vi "Write System.vi"(8 "error in (no error)":errorcluster, 10 "System":refnum<class "Message Enqueuer.lvclass">, 11 "Command in":refnum<class "Command Actor.lvclass">) -> (0 "error out":errorcluster, 3 "Command out":refnum<class "Command Actor.lvclass">)   [LabVIEW 2014, in "Robot Actor Framework.lvlib" / "Command Actor.lvlib" / "Command Actor.lvclass"]
uses:
  Command Actor.lvclass
  <vilib>/ActorFramework/Message Enqueuer/Message Enqueuer.lvclass
  Command Actor.lvclass/Command Actor.ctl
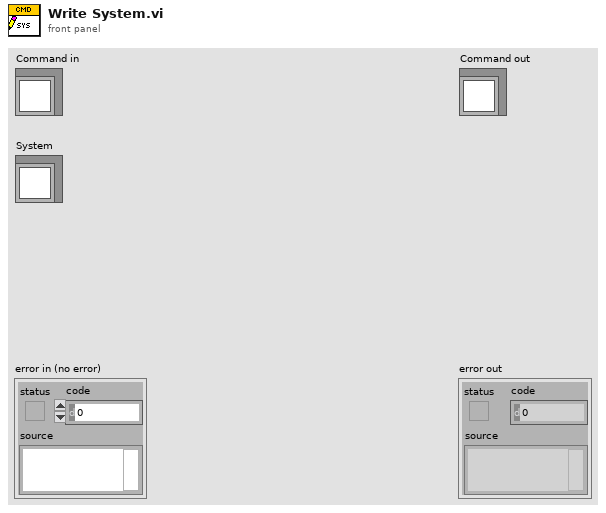
[diagram p1: front panel]
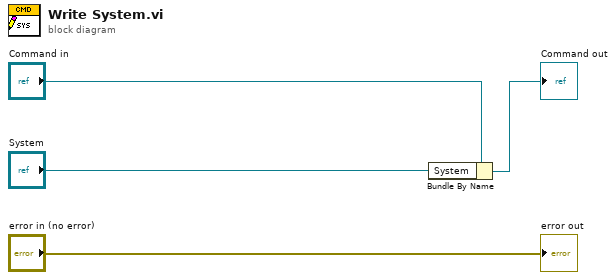
[diagram p0: block diagram]
diagram:
  n1 = Bundle By Name(cluster="Command in", "System"="System") -> (→"Command out":refnum<class "Command Actor.lvclass">)
  "error out" <- "error in (no error)"
